vi "MyRIO Controller.vi"() -> ()   [LabVIEW 2017]
doc: "The myRIO Project template acquires acceleration data from the onboard accelerometer and displays the changes of acceleration values in a waveform chart."
uses:
  <vilib>/myRIO/Instrument Drivers/Onboard IO/DIO/typedefs/DIO Reference.ctl
  <vilib>/myRIO/Common/Instrument Driver Framework/Utilities/typedefs/myRIO Generic Hardware Reference.ctl
  <vilib>/myRIO/Common/Instrument Driver Framework/Utilities/typedefs/Hardware Version Enum.ctl
  <vilib>/myRIO/Common/Instrument Driver Framework/Utilities/typedefs/myRIO v1.0 Reference.ctl
  <vilib>/myRIO/Common/Instrument Driver Framework/Utilities/typedefs/Generic FPGA Reference.ctl
  <vilib>/myRIO/Common/Instrument Driver Framework/myRIO v1.0/DIO/typedefs/DIO Channels List.ctl
  <vilib>/myRIO/Common/Instrument Driver Framework/myRIO v1.0/DIO/typedefs/DIO Channels Enum.ctl
  <vilib>/userdefined/High Color/nirio_resource_hc.ctl
  <vilib>/myRIO/Instrument Drivers/Onboard Devices/Accelerometer/typedefs/Accelerometer Reference.ctl
  <vilib>/myRIO/Common/Instrument Driver Framework/myRIO v1.0/Accelerometer/typedefs/Accelerometer Channels List.ctl
  <vilib>/myRIO/Common/Instrument Driver Framework/myRIO v1.0/Accelerometer/typedefs/Accelerometer Channels Enum.ctl
  <vilib>/myRIO/Instrument Drivers/Onboard IO/AI/typedefs/AI Reference.ctl
  <vilib>/myRIO/Common/Instrument Driver Framework/myRIO v1.0/AI/typedefs/AI Channels List.ctl
  <vilib>/myRIO/Common/Instrument Driver Framework/myRIO v1.0/AI/typedefs/AI Channels Enum.ctl
  <vilib>/myRIO/Common/Instrument Driver Framework/Utilities/typedefs/Analog Scaling Constants List.ctl
  <vilib>/myRIO/Common/Instrument Driver Framework/Utilities/typedefs/Analog Scaling Constants.ctl
  <vilib>/myRIO/Instrument Drivers/Onboard IO/PWM/typedefs/PWM Reference.ctl
  <vilib>/myRIO/Common/Instrument Driver Framework/myRIO v1.0/PWM/typedefs/PWM Channels Enum.ctl
  <vilib>/myRIO/Instrument Drivers/Onboard IO/PWM/typedefs/PWM Configuration.ctl
  <vilib>/myRIO/Common/Instrument Driver Framework/Utilities/vis/Is FPGA Ref Available.vi
  <vilib>/myRIO/Common/Instrument Driver Framework/myRIO v1.0/DIO/vis/myRIO v1.1 Open DIO.vi
  <vilib>/myRIO/Instrument Drivers/Onboard IO/DIO/vis/Write.vi
  <vilib>/myRIO/Instrument Drivers/Onboard IO/DIO/vis/Read.vi
  <vilib>/myRIO/Common/Instrument Driver Framework/myRIO v1.0/PWM/vis/myRIO v1.1 Open PWM.vi
  <vilib>/myRIO/Instrument Drivers/Onboard IO/PWM/vis/Set Duty Cycle and Frequency.vi
  <vilib>/myRIO/Common/Instrument Driver Framework/myRIO v1.0/AI/vis/myRIO v1.1 Open AI.vi
  <vilib>/myRIO/Instrument Drivers/Onboard IO/AI/vis/Read.vi
  <vilib>/myRIO/Common/Instrument Driver Framework/myRIO v1.0/Accelerometer/vis/myRIO v1.1 Open Accelerometer.vi
  <vilib>/myRIO/Instrument Drivers/Onboard Devices/Accelerometer/vis/Read.vi
  <vilib>/myRIO/Common/Instrument Driver Framework/Utilities/vis/Validate Channels.vi
  <vilib>/myRIO/Common/Instrument Driver Framework/myRIO v1.0/DIO/vis/myRIO v1.0 Reserve DIO.vi
  <vilib>/myRIO/Common/Instrument Driver Framework/myRIO v1.0/PWM/vis/myRIO v1.0 Reserve PWM.vi
  <vilib>/myRIO/Common/Instrument Driver Framework/myRIO v1.0/AI/vis/myRIO v1.0 Reserve AI.vi
  <vilib>/myRIO/Common/Instrument Driver Framework/myRIO v1.0/Accelerometer/vis/myRIO v1.0 Reserve Accelerometer.vi
  <vilib>/myRIO/Common/Instrument Driver Framework/myRIO v1.0/UART/vis/myRIO v1.0 Close UART.vi
  <vilib>/myRIO/Common/Instrument Driver Framework/myRIO v1.0/Resource Manager/vis/myRIO v1.0 Reserve Channel List.vi
  <vilib>/myRIO/Common/Instrument Driver Framework/myRIO v1.0/DIO/vis/myRIO v1.0 Build MUX Configuration DIO.vi
  <vilib>/myRIO/Common/Instrument Driver Framework/myRIO v1.0/PWM/vis/myRIO v1.0 Build MUX Configuration PWM.vi
  <vilib>/myRIO/Common/Instrument Driver Framework/myRIO v1.0/AI/vis/myRIO v1.0 Build MUX Configuration AI.vi
  <vilib>/myRIO/Common/Instrument Driver Framework/myRIO v1.0/Accelerometer/vis/myRIO v1.0 Build MUX Configuration Accelerometer.vi
  <vilib>/myRIO/Common/Instrument Driver Framework/myRIO v1.0/Resource Manager/vis/myRIO v1.0 Reserve Channel.vi
  <vilib>/myRIO/Common/Instrument Driver Framework/myRIO v1.0/Resource Manager/vis/myRIO v1.0 Unreserve Channel.vi
  <vilib>/myRIO/Common/Instrument Driver Framework/myRIO v1.0/Resource Manager/vis/myRIO v1.0 Create Configuration List.vi
  <vilib>/myRIO/Common/Instrument Driver Framework/myRIO v1.0/Resource Manager/vis/myRIO v1.0 Build Mutex Name.vi
  <vilib>/Utility/VariantDataType/GetNumericInfo.vi
  <vilib>/Utility/error.llb/Error Cluster From Error Code.vi
  <vilib>/myRIO/Common/Instrument Driver Framework/myRIO v1.0/myRIO v1.1 Open.vi
  <vilib>/myRIO/Common/Instrument Driver Framework/Utilities/vis/IO Manager.vi
  <vilib>/myRIO/Common/Instrument Driver Framework/Utilities/vis/Configuration Manager.vi
  <vilib>/myRIO/Common/Instrument Driver Framework/myRIO v1.0/Resource Manager/vis/myRIO v1.0 Configure IO.vi
  <vilib>/myRIO/Common/Instrument Driver Framework/myRIO v1.0/myRIO v1.0 Close.vi
  <vilib>/myRIO/Common/Instrument Driver Framework/myRIO v1.0/DIO/vis/myRIO v1.0 Write DIO.vi
  <vilib>/myRIO/Common/Instrument Driver Framework/myRIO v1.0/Accelerometer/vis/myRIO v1.0 Get Scaling Constant Accelerometer.vi
  <vilib>/myRIO/Common/Instrument Driver Framework/myRIO v1.0/Accelerometer/vis/myRIO v1.0 Read Accelerometer.vi
  <vilib>/myRIO/Common/Instrument Driver Framework/myRIO v1.0/AI/vis/myRIO v1.0 Get Scaling Constants AI.vi
  <vilib>/myRIO/Common/Instrument Driver Framework/myRIO v1.0/AI/vis/myRIO v1.0 Read AI.vi
  <vilib>/myRIO/Common/Instrument Driver Framework/myRIO v1.0/PWM/vis/myRIO v1.0 Write PWM.vi
  <vilib>/myRIO/Common/Instrument Driver Framework/myRIO v1.0/DIO/vis/myRIO v1.0 Read DIO.vi
  <vilib>/myRIO/Common/Instrument Driver Framework/Utilities/vis/FPGA Ref Manager.vi
  <vilib>/myRIO/Common/Instrument Driver Framework/myRIO v1.0/myRIO v1.0 Reset FPGA.vi
  <vilib>/myRIO/Common/Instrument Driver Framework/myRIO v1.0/IRQ/vis/myRIO v1.0 IRQ Info FGV.vi
  <vilib>/myRIO/Common/Instrument Driver Framework/myRIO v1.0/IRQ/vis/myRIO v1.0 Timer IRQ Info FGV.vi
  <vilib>/myRIO/Common/Instrument Driver Framework/myRIO v1.0/IRQ/vis/myRIO v1.0 ISR Agent.vi
  <vilib>/myRIO/Express VI/Onboard Devices/LED/LED Express VI.xnode
  <vilib>/myRIO/Instrument Drivers/Onboard IO/DIO/vis/myRIO DIO Open.xnode
  <vilib>/myRIO/Express VI/Onboard Devices/Accelerometer/Accelerometer Express VI.xnode
  <vilib>/myRIO/Instrument Drivers/Onboard Devices/Accelerometer/vis/myRIO Accelerometer Open.xnode
  <vilib>/myRIO/Express VI/Onboard IO/AI/AI Express VI.xnode
  <vilib>/myRIO/Instrument Drivers/Onboard IO/AI/vis/myRIO AI Open.xnode
  <vilib>/myRIO/Express VI/Onboard IO/PWM/PWM Express VI.xnode
  <vilib>/myRIO/Instrument Drivers/Onboard IO/PWM/vis/myRIO PWM Open.xnode
  <vilib>/myRIO/Express VI/Onboard Devices/Button/Button Express VI.xnode
  <vilib>/myRIO/Instrument Drivers/Utilities/Utilities.lvlib
  <vilib>/myRIO/Instrument Drivers/Onboard Devices/Accelerometer/Accelerometer.lvlib
  <vilib>/myRIO/Instrument Drivers/Onboard IO/AI/AI.lvlib
  <vilib>/myRIO/Instrument Drivers/Onboard IO/PWM/PWM.lvlib
  <vilib>/myRIO/Instrument Drivers/Onboard IO/DIO/DIO.lvlib
panel:
  out "Cooling":bool
  out "Countdown timer":dbl format="%#_4g"
  out "Movement":bool
  in  "Max Movement":u8
  in  "Max temp":i8
  out "Bytes sent":dbl
  out "Send to PC":i8
  out "Temp":dbl format="%#_4g"
  out "Local":bool
  out "Input from PC":dbl
  out "Cluster sent":T1 {"Code sent" format="%#_4g"; "Z" format="%#_4g"; "Y" format="%#_4g"; "X" format="%#_4g"; "Core Temp" format="%#_4g"}
  in  "Stop":bool
  out "Acceleration":T2(graph)
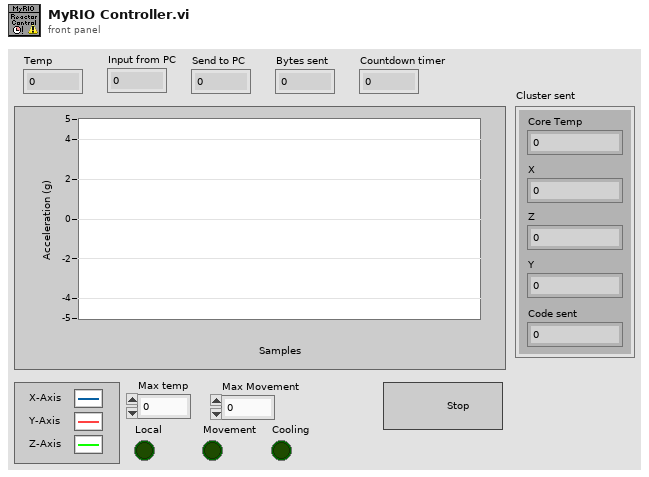
[diagram p1: front panel]
types:
  T1 = cluster{"Core Temp":dbl, "X":dbl, "Y":dbl, "Z":dbl, "Code sent":dbl}
  T2 = cluster{"X-Axis":dbl, "Y-Axis":dbl, "Z-Axis":dbl}
  T3 = typedef "DIO.lvlib/DIO Reference.ctl" = cluster{"myRIO Reference":T4, "DIO Channels List":T8}
  T4 = typedef "myRIO Generic Hardware Reference.ctl" = cluster{"myRIO Model":T5, "myRIO Hardware Reference":T6}
  T5 = typedef "Hardware Version Enum.ctl" = enum16{"Unknown", "myRIO-1900", "myRIO-1950", "roboRIO", "NI ELVIS RIO CM"}
  T6 = typedef "myRIO v1.0 Reference.ctl" = cluster{"Generic FPGA Reference":T7, "Allow multiple opens":bool}
  T7 = typedef "Generic FPGA Reference.ctl" = refnum<k20>
  T8 = typedef "DIO Channels List.ctl" = T9[]
  T9 = typedef "DIO Channels Enum.ctl" = enum16{"Not Connected", "C/DIO0", "C/DIO1", "C/DIO2", "C/DIO3", "C/DIO4", "C/DIO5", "C/DIO6", "C/DIO7", "A/DIO0", "A/DIO1", "A/DIO2", "A/DIO3", "A/DIO4", "A/DIO5", "A/DIO6", "A/DIO7", "A/DIO8", "A/DIO9", "A/DIO10", "A/DIO11", "A/DIO12", "A/DIO13", "A/DIO14", "A/DIO15", "B/DIO0", "B/DIO1", "B/DIO2", "B/DIO3", "B/DIO4", "B/DIO5", "B/DIO6", "B/DIO7", "B/DIO8", "B/DIO9", "B/DIO10", "B/DIO11", "B/DIO12", "B/DIO13", "B/DIO14", "B/DIO15", "LED0", "LED1", "LED2", "LED3", "Button0", "DIO/DIO0", "DIO/DIO1", "DIO/DIO2", "DIO/DIO3", "DIO/DIO4", "DIO/DIO5", "DIO/DIO6", "DIO/DIO7", "DIO/DIO8", "DIO/DIO9", "SPI/CS0", "SPI/CS1", "SPI/CS2", "SPI/CS3", "LED RADIO (Green)", "LED RADIO (Red)", "LED COMM (Green)", "LED COMM (Red)", "LED MODE (Green)", "LED MODE (Red)"}
  T10 = typedef "nirio_resource_hc.ctl" = tag
  T11 = typedef "PWM.lvlib/PWM Reference.ctl" = cluster{"myRIO Reference":T4, "PWM Channels Enum":T12, "PWM Configuration":T13}
  T12 = typedef "PWM Channels Enum.ctl" = enum16{"Not Connected", "C/PWM0", "C/PWM1", "A/PWM0", "A/PWM1", "A/PWM2", "B/PWM0", "B/PWM1", "B/PWM2", "PWM/PWM0", "PWM/PWM1", "PWM/PWM2", "PWM/PWM3", "PWM/PWM4", "PWM/PWM5", "PWM/PWM6", "PWM/PWM7", "PWM/PWM8", "PWM/PWM9"}
  T13 = typedef "PWM.lvlib/PWM Configuration.ctl" = cluster{"Frequency":dbl, "Duty Cycle":dbl}
  T14 = typedef "AI.lvlib/AI Reference.ctl" = cluster{"myRIO Reference":T4, "AI Channels List":T15, "AI Scaling Constants List":T17}
  T15 = typedef "AI Channels List.ctl" = T16[]
  T16 = typedef "AI Channels Enum.ctl" = enum16{"Not Connected", "AudioIn/Left", "AudioIn/Right", "C/AI0", "C/AI1", "A/AI0", "A/AI1", "A/AI2", "A/AI3", "B/AI0", "B/AI1", "B/AI2", "B/AI3", "AI/AI0", "AI/AI1", "AI/AI2", "AI/AI3"}
  T17 = typedef "Analog Scaling Constants List.ctl" = T18[]
  T18 = typedef "Analog Scaling Constants.ctl" = cluster{"LSB Weight (Volts)":dbl, "Offset (Volts)":dbl, "Signed?":bool}
  T19 = typedef "Accelerometer.lvlib/Accelerometer Reference.ctl" = cluster{"myRIO Reference":T4, "Accelerometer Channels List":T20, "LSB Weight":dbl}
  T20 = typedef "Accelerometer Channels List.ctl" = T21[]
  T21 = typedef "Accelerometer Channels Enum.ctl" = enum16{"Not Connected", "X-Axis", "Y-Axis", "Z-Axis"}
  T22 = cluster{dbl, "X-Axis":dbl, "Y-Axis":dbl, dbl, "Send to PC":i8}
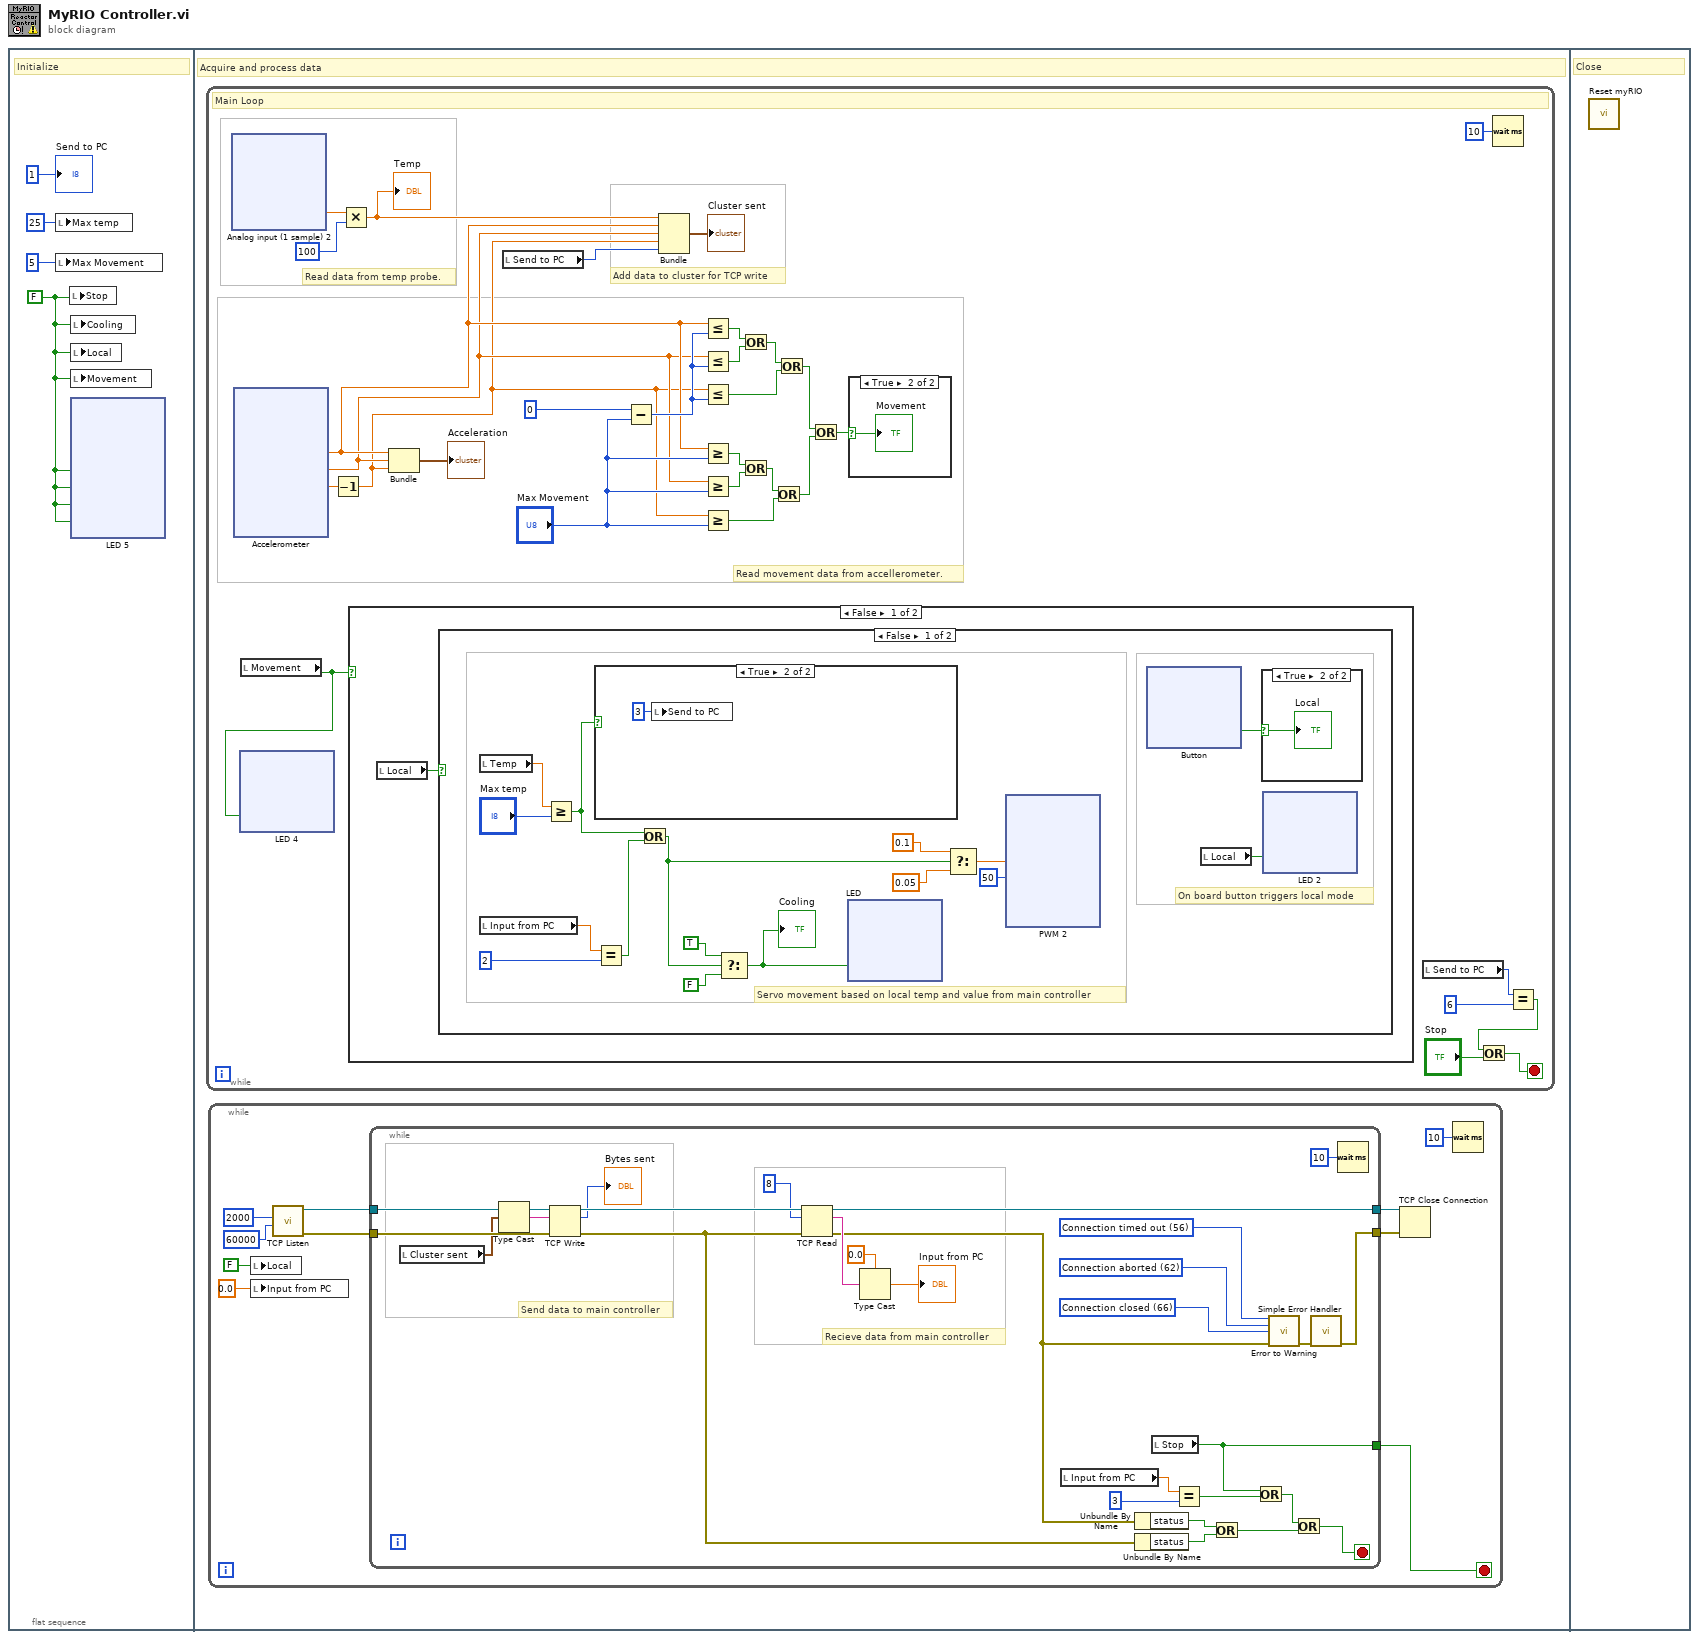
[diagram p0: block diagram]
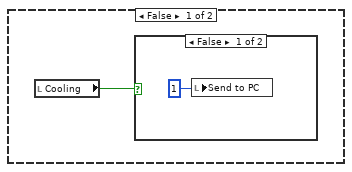
[diagram p3: hidden frame]
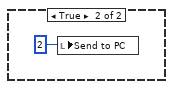
[diagram p4: hidden frame]
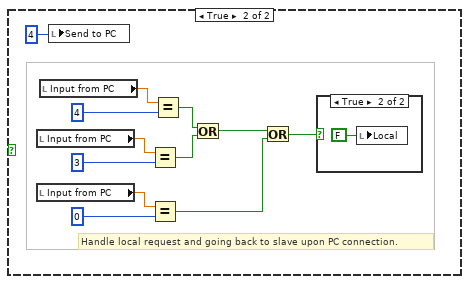
[diagram p5: hidden frame]
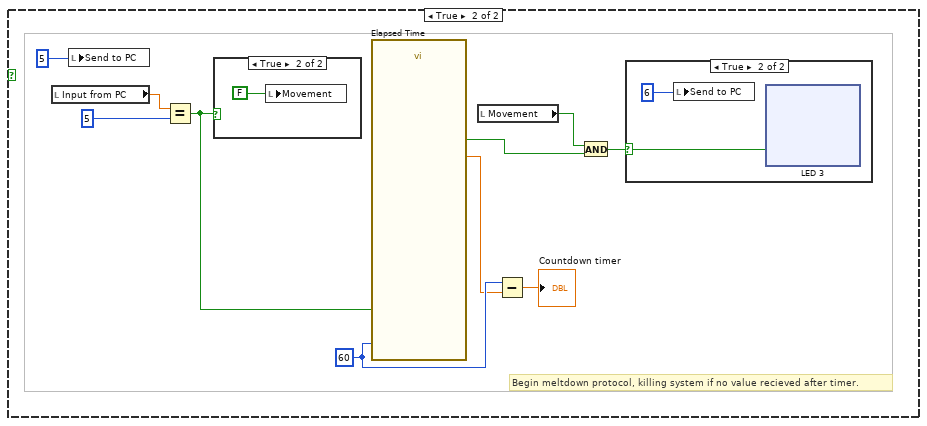
[diagram p7: hidden frame]
diagram:
  n1 = flat-sequence {
    frame #0 {
      w1 = FALSE
      # "Initialize"
      n2 = local write "Max temp"(25) -> ()
      n3 = local write "Max Movement"(5) -> ()
      n4 = local write "Stop"(w1) -> ()
      n5 = local write "Cooling"(w1) -> ()
      n6 = local write "Local"(w1) -> ()
      n7 = local write "Movement"(w1) -> ()
      n8 = xnode "LED 5"("LED0"=w1, "LED1"=w1, "LED2"=w1, "LED3"=w1) -> ()  [unwired: 1 in, 1 out]
      "Send to PC" <- 1
    }
    frame #1 {
      # "Acquire and process data"
      n9 = while {
        stop <- w85 stop-if-true
        # "Add data to cluster for TCP write"
        # "Read data from temp probe."
        # "Read movement data from accellerometer."
        # "Main Loop"
        n10 = xnode "Analog input (1 sample) 2"() -> ("A/AI3 (Pin 9)"=w109:dbl)  [unwired: 1 in, 1 out]
        n11 = xnode "Accelerometer"() -> ("X-Axis"=w90:dbl, "Y-Axis"=w89:dbl, "Z-Axis"=w107:dbl)  [unwired: 1 in, 1 out]
        n12 = local read "Movement"() -> (w86:bool)
        n13 = xnode "LED 4"("LED2"=w86) -> ()  [unwired: 1 in, 1 out]
        n14 = Decrement(x=w107) -> (x-1=w88:dbl)
        n15 = Multiply(x=w109, y=100) -> (x*y=w105:dbl)
        "Temp" <- w105
        n16 = case shown="False" w86 {
          frame False {
            n17 = local read "Local"() -> (w147:bool)
            n18 = case shown="False" w147 {
              frame False {
                # "On board button triggers local mode"
                # "Servo movement based on local temp and value from main controller"
                n19 = local read "Temp"() -> (w160:dbl)
                n20 = local read "Input from PC"() -> (w159:dbl)
                n21 = Greater Or Equal?(x=w160, y="Max temp") -> (x >= y?=w161:bool)
                n22 = case shown="True" w161 {
                  frame False {
                    n23 = local read "Cooling"() -> (w235:bool)
                    n24 = case shown="False" w235 {
                      frame False {
                        n25 = local write "Send to PC"(1) -> ()
                      }
                      frame True {
                        n26 = local write "Send to PC"(2) -> ()
                      }
                    }
                  }
                  frame True {
                    n27 = local write "Send to PC"(3) -> ()
                  }
                }
                n28 = Equal?(x=w159, y=2) -> (x = y?=w157:bool)
                n29 = Or(x=w161, y=w157) -> (x .or. y?=w158:bool)
                n30 = Select(t=TRUE, s=w158, f=FALSE) -> (s? t:f=w163:bool)
                "Cooling" <- w163
                n31 = xnode "LED"("LED0"=w163) -> ()  [unwired: 1 in, 1 out]
                n32 = Select(t=0.1, s=w158, f=0.05) -> (s? t:f=w162:dbl)
                n33 = xnode "PWM 2"("Duty Cycle"=w162, "Frequency [Hz]"=50) -> ()  [unwired: 1 in, 1 out]
                n34 = xnode "Button"() -> ("Value"=w149:bool)  [unwired: 1 in, 1 out]
                n35 = local read "Local"() -> (w148:bool)
                n36 = case shown="True" w149 {
                  selector: w149 -> [_ w199]
                  frame False {
                  }
                  frame True {
                    "Local" <- w199
                  }
                }
                n37 = xnode "LED 2"("LED1"=w148) -> ()  [unwired: 1 in, 1 out]
              }
              frame True {
                # "Handle local request and going back to slave upon PC connection."
                n38 = local read "Input from PC"() -> (w319:dbl)
                n39 = local read "Input from PC"() -> (w310:dbl)
                n40 = local read "Input from PC"() -> (w318:dbl)
                n41 = local write "Send to PC"(4) -> ()
                n42 = Equal?(x=w319, y=3) -> (x = y?=w314:bool)
                n43 = Equal?(x=w310, y=0) -> (x = y?=w309:bool)
                n44 = Equal?(x=w318, y=4) -> (x = y?=w315:bool)
                n45 = Or(x=w315, y=w314) -> (x .or. y?=w312:bool)
                n46 = Or(x=w312, y=w309) -> (x .or. y?=w313:bool)
                n47 = case shown="True" w313 {
                  frame False {
                  }
                  frame True {
                    n48 = local write "Local"(FALSE) -> ()
                  }
                }
              }
            }
          }
          frame True {
            w325 = 60
            # "Begin meltdown protocol, killing system if no value recieved after timer."
            n49 = local read "Input from PC"() -> (w329:dbl)
            n50 = local write "Send to PC"(5) -> ()
            n51 = Equal?(x=w329, y=5) -> (x = y?=w324:bool)
            n52 = case shown="True" w324 {
              frame False {
              }
              frame True {
                n53 = local write "Movement"(FALSE) -> ()
              }
            }
            n54 = call "Elapsed Time"("Time Target (s)"=w325, "Reset"=w324) -> ("Elapsed Time (s)"=w322:dbl, "Time has Elapsed"=w326:bool)  [unwired: 10 in, 6 out]
            n55 = local read "Movement"() -> (w327:bool)
            n56 = Subtract(x=w325, y=w322) -> (x-y=→"Countdown timer":dbl)
            n57 = And(x=w327, y=w326) -> (x .and. y?=w328:bool)
            n58 = case shown="True" w328 {
              selector: w328 -> [_ w332]
              frame False {
              }
              frame True {
                n59 = local write "Send to PC"(6) -> ()
                n60 = xnode "LED 3"("LED3"=w332) -> ()  [unwired: 1 in, 1 out]
              }
            }
          }
        }
        n61 = Bundle("X-Axis"=w90, "Y-Axis"=w89, w88) -> (→"Acceleration":cluster{"X-Axis":dbl, "Y-Axis":dbl, dbl})  [unwired: 1 in]
        n62 = local read "Send to PC"() -> (w104:i8)
        n63 = Subtract(x=0, y="Max Movement") -> (x-y=w91:i32)
        n64 = Bundle(w105, "X-Axis"=w90, "Y-Axis"=w89, w88, "Send to PC"=w104) -> (→"Cluster sent":T22)  [unwired: 1 in]
        n65 = Less Or Equal?(x=w90, y=w91) -> (x <= y?=w102:bool)
        n66 = Less Or Equal?(x=w89, y=w91) -> (x <= y?=w101:bool)
        n67 = Less Or Equal?(x=w88, y=w91) -> (x <= y?=w99:bool)
        n68 = Greater Or Equal?(x=w90, y="Max Movement") -> (x >= y?=w98:bool)
        n69 = Greater Or Equal?(x=w89, y="Max Movement") -> (x >= y?=w97:bool)
        n70 = Greater Or Equal?(x=w88, y="Max Movement") -> (x >= y?=w96:bool)
        n71 = Or(x=w102, y=w101) -> (x .or. y?=w100:bool)
        n72 = Or(x=w98, y=w97) -> (x .or. y?=w95:bool)
        n73 = Or(x=w95, y=w96) -> (x .or. y?=w94:bool)
        n74 = Or(x=w100, y=w99) -> (x .or. y?=w93:bool)
        n75 = Or(x=w93, y=w94) -> (x .or. y?=w87:bool)
        n76 = case shown="True" w87 {
          selector: w87 -> [_ w370]
          frame False {
          }
          frame True {
            "Movement" <- w370
          }
        }
        n77 = local read "Send to PC"() -> (w83:i8)
        n78 = Wait (ms)(milliseconds to wait=u32 10) -> ()  [unwired: 1 out]
        n79 = Equal?(x=w83, y=6) -> (x = y?=w81:bool)
        n80 = Or(x=w81, y="Stop") -> (x .or. y?=w85:bool)
      }
      n81 = while {
        stop <- w43 stop-if-true
        n82 = local write "Local"(FALSE) -> ()
        n83 = local write "Input from PC"(0.0) -> ()
        n84 = call <vilib>:"TCP Listen.vi"("timeout ms (wait forever: -1)"=60000, "port"=2000) -> ("error out"=w52:errorcluster, "connection ID"=w51:refnum<k5>)  [unwired: 5 in, 3 out]
        n85 = while {
          tunnel: w51 -> [w80]
          tunnel: w52 -> [w79]
          tunnel: [w75] -> w47
          tunnel: [w61] -> w46
          tunnel: [w53] -> w43
          stop <- w66 stop-if-true
          w58 = 66 items=["No Error", "Argument Error", "Memory Full", "Out of Zone", "End of File", "File Already Open", "Generic File IO Error", "File Not Found", "File Permission Error", "Disk Full", "Duplicate Path", "Too Many Files Open", "Not Enabled", "Resource File Not Found", "Cannot Add Resource", "Resource Not Found", "Image Not Found", "Image Memory Error", "Pen Does Not Exist", "Config Bad Type", "Config Token Not Found", "Config Parse Error", "Config Memory Error", "Bad External Code Format", "Bad External Code Offset", "External Code Not Present", "Null Window", "Destroy Window Mixup", "Null Menu", "Print Aborted", "Bad Print Record", "Print Driver Error", "Windows Error During Print", "Memory Error During Print", "Print Dialog Error", "Generic Print Error", "Invalid Device Refnum", "Device Not Found", "Device Parameter Error", "Device Unit Error", "Can't Open Device", "Device Call Aborted", "Generic Error", "Cancelled By User", "Object ID Too Low", "Object ID Too High", "Object Not In Heap", "Unknown Heap", "Bad DefProc ID", "DefProc Not In Table", "Message Out Of Range", "Null Method", "Unknown Message", "Manager Call Not Supported", "Bad address", "Connection In progress", "Connection timed out", "Connection is already in progress", "Network attribute not supported", "Network error", "Address in use", "System out of memory", "Connection aborted", "Connection refused", "Connection is not connected", "Connection is already connected", "Connection closed", "Initialize error (interapplication manager)", "Bad occurrence", "Wait on unbound occurrence handler", "Occurrence queue overflow", "Bad path", "Semaphore not signaled", "Unrecognized type (interapplication manager)"] ("1st Error to Convert")
          w59 = 62 items=["No Error", "Argument Error", "Memory Full", "Out of Zone", "End of File", "File Already Open", "Generic File IO Error", "File Not Found", "File Permission Error", "Disk Full", "Duplicate Path", "Too Many Files Open", "Not Enabled", "Resource File Not Found", "Cannot Add Resource", "Resource Not Found", "Image Not Found", "Image Memory Error", "Pen Does Not Exist", "Config Bad Type", "Config Token Not Found", "Config Parse Error", "Config Memory Error", "Bad External Code Format", "Bad External Code Offset", "External Code Not Present", "Null Window", "Destroy Window Mixup", "Null Menu", "Print Aborted", "Bad Print Record", "Print Driver Error", "Windows Error During Print", "Memory Error During Print", "Print Dialog Error", "Generic Print Error", "Invalid Device Refnum", "Device Not Found", "Device Parameter Error", "Device Unit Error", "Can't Open Device", "Device Call Aborted", "Generic Error", "Cancelled By User", "Object ID Too Low", "Object ID Too High", "Object Not In Heap", "Unknown Heap", "Bad DefProc ID", "DefProc Not In Table", "Message Out Of Range", "Null Method", "Unknown Message", "Manager Call Not Supported", "Bad address", "Connection In progress", "Connection timed out", "Connection is already in progress", "Network attribute not supported", "Network error", "Address in use", "System out of memory", "Connection aborted", "Connection refused", "Connection is not connected", "Connection is already connected", "Connection closed", "Initialize error (interapplication manager)", "Bad occurrence", "Wait on unbound occurrence handler", "Occurrence queue overflow", "Bad path", "Semaphore not signaled", "Unrecognized type (interapplication manager)"] ("1st Error to Convert")
          w60 = 56 items=["No Error", "Argument Error", "Memory Full", "Out of Zone", "End of File", "File Already Open", "Generic File IO Error", "File Not Found", "File Permission Error", "Disk Full", "Duplicate Path", "Too Many Files Open", "Not Enabled", "Resource File Not Found", "Cannot Add Resource", "Resource Not Found", "Image Not Found", "Image Memory Error", "Pen Does Not Exist", "Config Bad Type", "Config Token Not Found", "Config Parse Error", "Config Memory Error", "Bad External Code Format", "Bad External Code Offset", "External Code Not Present", "Null Window", "Destroy Window Mixup", "Null Menu", "Print Aborted", "Bad Print Record", "Print Driver Error", "Windows Error During Print", "Memory Error During Print", "Print Dialog Error", "Generic Print Error", "Invalid Device Refnum", "Device Not Found", "Device Parameter Error", "Device Unit Error", "Can't Open Device", "Device Call Aborted", "Generic Error", "Cancelled By User", "Object ID Too Low", "Object ID Too High", "Object Not In Heap", "Unknown Heap", "Bad DefProc ID", "DefProc Not In Table", "Message Out Of Range", "Null Method", "Unknown Message", "Manager Call Not Supported", "Bad address", "Connection In progress", "Connection timed out", "Connection is already in progress", "Network attribute not supported", "Network error", "Address in use", "System out of memory", "Connection aborted", "Connection refused", "Connection is not connected", "Connection is already connected", "Connection closed", "Initialize error (interapplication manager)", "Bad occurrence", "Wait on unbound occurrence handler", "Occurrence queue overflow", "Bad path", "Semaphore not signaled", "Unrecognized type (interapplication manager)"] ("1st Error to Convert")
          # "Recieve data from main controller"
          # "Send data to main controller"
          n86 = local read "Cluster sent"() -> (w76:T1)
          n87 = Type Cast(x=w76) -> (*(type *) &x=w78:string)  [unwired: 1 in]
          n88 = TCP Write(connection ID=w80, data in=w78, error in (no error)=w79) -> (connection ID out=w73:refnum<k5>, bytes written=→"Bytes sent":i32, error out=w74:errorcluster)  [unwired: 1 in]
          n89 = TCP Read(connection ID=w73, bytes to read=8, error in (no error)=w74) -> (connection ID out=w75:refnum<k5>, data out=w71:string, error out=w63:errorcluster)  [unwired: 2 in]
          n90 = Type Cast(type=0.0, x=w71) -> (*(type *) &x=→"Input from PC":dbl)
          n91 = local read "Input from PC"() -> (w57:dbl)
          n92 = Unbundle By Name(w63) -> ("status"=w70:bool)
          n93 = Unbundle By Name(w74) -> ("status"=w69:bool)
          n94 = local read "Stop"() -> (w53:bool)
          n95 = Equal?(x=w57, y=3) -> (x = y?=w55:bool)
          n96 = Or(x=w70, y=w69) -> (x .or. y?=w65:bool)
          n97 = Or(x=w53, y=w55) -> (x .or. y?=w54:bool)
          n98 = call <vilib>:"Error to Warning.vi"("1st Error to Convert"=w60, "2nd Error to Convert"=w59, "3rd Error to Convert"=w58, "error in"=w63) -> ("warning out"=w62:errorcluster)  [unwired: 2 in, 9 out]
          n99 = Or(x=w54, y=w65) -> (x .or. y?=w66:bool)
          n100 = call <vilib>:"Simple Error Handler.vi"("error in (no error)"=w62) -> ("error out"=w61:errorcluster)  [unwired: 4 in, 4 out]
          n101 = Wait (ms)(milliseconds to wait=u32 10) -> ()  [unwired: 1 out]
        }
        n102 = TCP Close Connection(connection ID=w47, error in (no error)=w46) -> ()  [unwired: 1 in, 2 out]
        n103 = Wait (ms)(milliseconds to wait=u32 10) -> ()  [unwired: 1 out]
      }
    }
    frame #2 {
      # "Close"
      n104 = call <vilib>:"Reset myRIO.vi"() -> ()  [unwired: 11 in, 1 out]
    }
  }
